vi "FIFO Bucket Challenge.vi"() -> ()   [LabVIEW 2010]
doc: "This VI demonstrates how elements are written to and read from a Target-Scoped FIFO on FPGA. When the user selects write, elements will be written to the FIFO in increasing order. If the FIFO runs out of room to write the data, the FIFO Full LED will become true. When the user selects to read from the FIFO, a different loop will begin to read from the FIFO one element at a time and the element will be displayed in the Element Read indicator. If the FIFO runs out of elements to read, the FIFO Empty LED will become true. The bucket is used to keep track of how many elements are currently in the FIFO. This number is calculated by taking the number of successful writes to the FIFO and subtracting the number of successful reads."
uses:
  <vilib>/rvi/LocalResourceManager/LocalResourceManager.xnode
  <vilib>/rvi/DataTransferAndStorage/Container/Common/niFpgaContainerState.ctl
  <vilib>/rvi/DataTransferAndStorage/Container/Common/niFpgaDataTypeControl.ctl
  <vilib>/rvi/DataTransferAndStorage/Container/Common/niFpgaContainerImplementationControl.ctl
  <vilib>/rvi/DataTransferAndStorage/Container/Common/niFpgaContainerArbitrationOptionsControl.ctl
  <vilib>/rvi/DataTransferAndStorage/Container/Common/niFpgaTransferTypeControl.ctl
  <vilib>/rvi/DataTransferAndStorage/Container/Common/niFpgaContainerInitializationParameters.ctl
  <vilib>/rvi/Memory/Memory_Types/niFpgaMemoryInterfaceConfiguration.ctl
  <vilib>/rvi/FIFO/Fifo_Types/niFpgaFifoControlLogicControl.ctl
  <vilib>/rvi/DataTransferAndStorage/Container/Common/niFpgaContainerMetaDataKey.ctl
  <vilib>/rvi/DataTransferAndStorage/Container/XNode/niFpgaContainer.xnode
  <vilib>/rvi/DataTransferAndStorage/Container/Common/niFpgaContainerGetUniqueNameForEmu.vi
  <vilib>/rvi/DataTransferAndStorage/Container/Common/niFpgaContainerSetEmuInfo.vi
  <vilib>/rvi/eio/common/nirviEmuReportErrorAndStop.vi
  <vilib>/rvi/FIFO/Fifo_Resource/nirvififoEmulationSetSize.vi
panel:
  out "Element Read":u16
  out "FIFO Empty":bool
  out "FIFO Full":bool
  out "# of writes":u16
  out "# of reads":u16
  out "Bucket":u16(slide) scale=0.0..36.0
  in  "Read":bool
  in  "Write":bool
  # "This VI demonstrates how elements are written to \nand read from a Target-Scoped FIFO on FPGA. \nPress write to write elements to the FPGA FIFO\nand read to read elemtnes off of the FPGA FIFO.\nThe bucket indicator shows how many elements\nare in the FPGA."
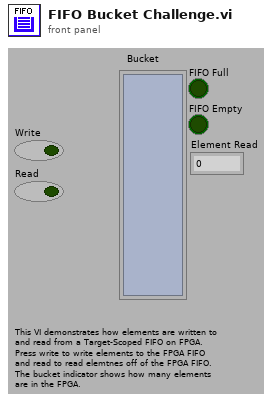
[diagram p1: front panel]
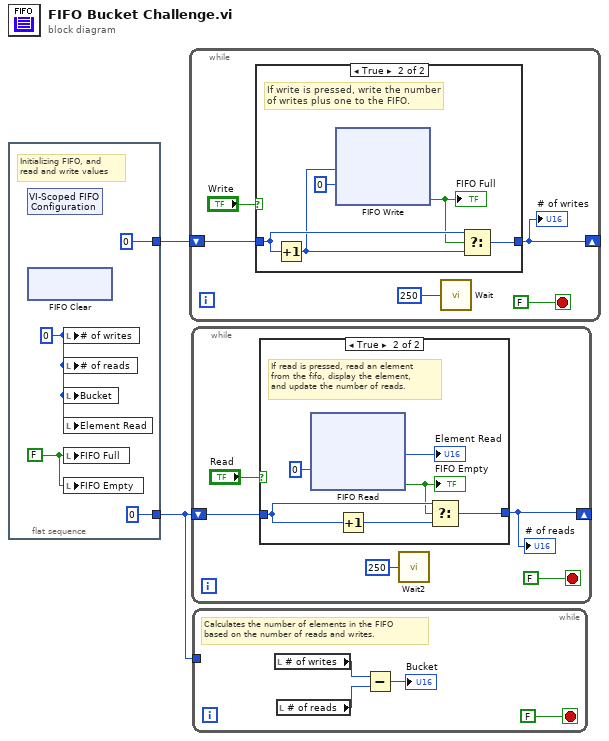
[diagram p0: block diagram]
diagram:
  n1 = flat-sequence {
    tunnel: [u16 0] -> w2
    tunnel: [u16 0] -> w1
    frame #0 {
      w4 = FALSE ("FIFO Full")
      w3 = u16 0 ("writes")
      # "Initializing FIFO, and\nread and write values"
      n2 = xnode "VI-Scoped FIFO Configuration"() -> ()  [unwired: 1 out]
      n3 = xnode ("FIFO Clear")() -> ()  [unwired: 1 in, 1 out]
      n4 = local write "# of writes"(w3) -> ()
      n5 = local write "# of reads"(w3) -> ()
      n6 = local write "Bucket"(w3) -> ()
      n7 = local write "Element Read"(w3) -> ()
      n8 = local write "FIFO Full"(w4) -> ()
      n9 = local write "FIFO Empty"(w4) -> ()
    }
  }
  n10 = while {
    shift-right: [w70] -> _
    shift-left: w2 -> [w73]
    stop <- FALSE stop-if-true
    n11 = case shown="True" "Write" {
      tunnel: w73 -> [w75 w79]
      tunnel: [w75 w80] -> w70
      frame False {
        # "If write is not pressed, do not \nupdate the number of writes."
      }
      frame True {
        # "If write is pressed, write the number\nof writes plus one to the FIFO."
        n12 = Increment(x=w79) -> (x+1=w78:u16)
        n13 = xnode ("FIFO Write")("Element"=w78, "Timeout"=0) -> ("Timed Out?"=w76:bool)  [unwired: 1 in, 1 out]
        "FIFO Full" <- w76
        n14 = Select(t=w79, s=w76, f=w78) -> (s? t:f=w80:u16)
      }
    }
    "# of writes" <- w70
    n15 = call "Wait"("Count(mSec)"=u32 250) -> ()  [unwired: 1 out]
  }
  n16 = while {
    shift-right: [w132] -> _
    shift-left: w1 -> [w135]
    stop <- FALSE stop-if-true
    n17 = case shown="True" "Read" {
      tunnel: w135 -> [w137 w142]
      tunnel: [w137 w141] -> w132
      frame False {
        # "If read is not pressed, do not \nupdate the number of reads."
      }
      frame True {
        # "If read is pressed, read an element\nfrom the fifo, display the element,\nand update the number of reads."
        n18 = xnode ("FIFO Read")("Timeout"=0) -> ("Element"=→"Element Read":i16, "Timed Out?"=w139:bool)  [unwired: 1 in, 1 out]
        "FIFO Empty" <- w139
        n19 = Increment(x=w142) -> (x+1=w143:u16)
        n20 = Select(t=w142, s=w139, f=w143) -> (s? t:f=w141:u16)
      }
    }
    "# of reads" <- w132
    n21 = call "Wait2"("Count(mSec)"=u32 250) -> ()  [unwired: 1 out]
  }
  n22 = while {
    tunnel: w1 -> [_]
    stop <- FALSE stop-if-true
    # "Calculates the number of elements in the FIFO\nbased on the number of reads and writes."
    n23 = local read "# of writes"() -> (w198:u16)
    n24 = local read "# of reads"() -> (w197:u16)
    n25 = Subtract(x=w198, y=w197) -> (x-y=→"Bucket":u16)
  }
